vi "Filter And List Splitters.vi"(8 "Error In":errorcluster, 10 "Splitter Refs":refnum<vi>[](array[refnum]), 11 "Control Reference Lists In":T1) -> (0 "Error Out":errorcluster, 3 "Control Reference Lists Out":T1)   [LabVIEW 2021, in "Appearance Actor.lvlib" / "Appearance Actor.lvclass"]
uses:
  Appearance Actor.lvclass
  Typedefs/Control Reference Lists--cluster.ctl
  Typedefs/Control Reference Lists-TitleBar--cluster.ctl
  Typedefs/Control Reference Lists-SideMenu--cluster.ctl
  Typedefs/Control Reference Lists-BodyPane--cluster.ctl
  Typedefs/Control Reference Lists-StatusBar--cluster.ctl
  <vilib>/regexp/Match Regular Expression.xnode
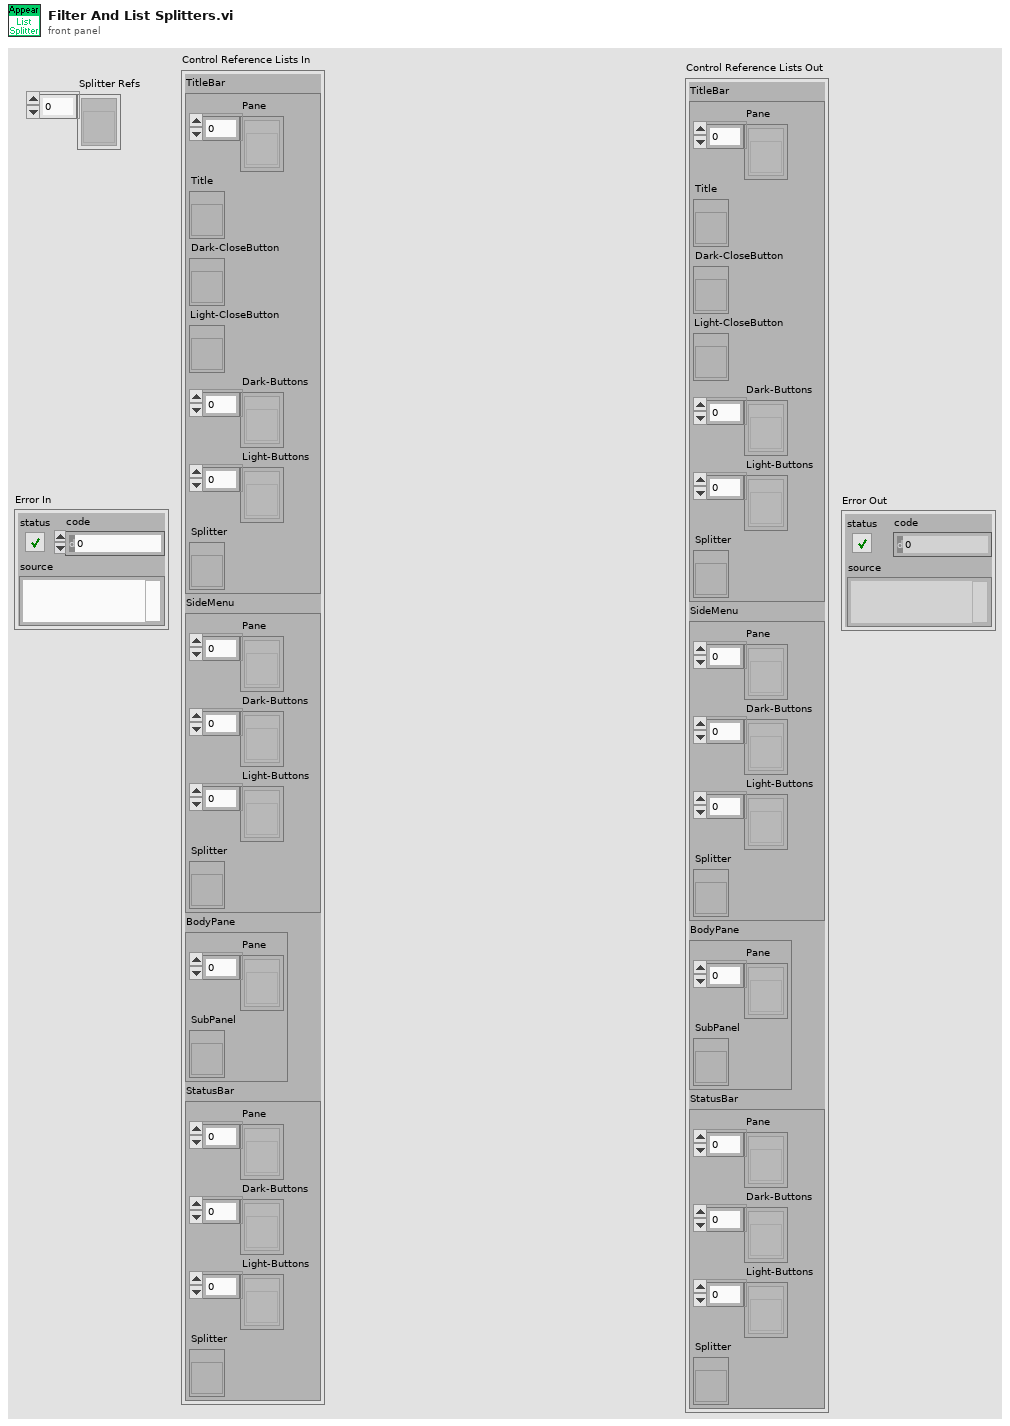
[diagram p1: front panel]
types:
  T1 = typedef "Control Reference Lists--cluster.ctl" = cluster{"TitleBar":T2, "SideMenu":T3, "BodyPane":T4, "StatusBar":T5}
  T2 = typedef "Control Reference Lists-TitleBar--cluster.ctl" = cluster{"Pane":refnum<vi>[], "Title":refnum<vi>, "Dark-CloseButton":refnum<vi>, "Light-CloseButton":refnum<vi>, "Dark-Buttons":refnum<vi>[], "Light-Buttons":refnum<vi>[], "Splitter":refnum<vi>}
  T3 = typedef "Control Reference Lists-SideMenu--cluster.ctl" = cluster{"Pane":refnum<vi>[], "Dark-Buttons":refnum<vi>[], "Light-Buttons":refnum<vi>[], "Splitter":refnum<vi>}
  T4 = typedef "Control Reference Lists-BodyPane--cluster.ctl" = cluster{"Pane":refnum<vi>[], "SubPanel":refnum<vi>}
  T5 = typedef "Control Reference Lists-StatusBar--cluster.ctl" = cluster{"Pane":refnum<vi>[], "Dark-Buttons":refnum<vi>[], "Light-Buttons":refnum<vi>[], "Splitter":refnum<vi>}
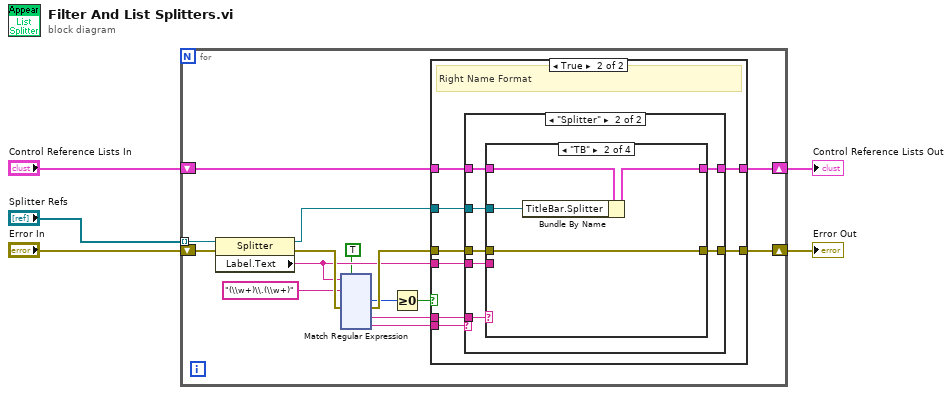
[diagram p0: block diagram]
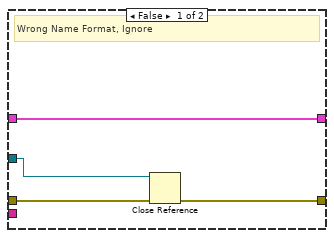
[diagram p2: hidden frame]
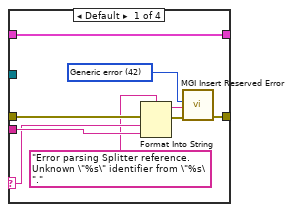
[diagram p4: hidden frame]
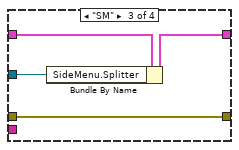
[diagram p5: hidden frame]
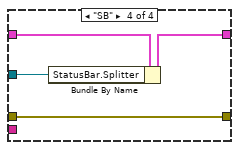
[diagram p6: hidden frame]
diagram:
  n1 = for {
    tunnel: "Splitter Refs" -> [w20] mode=indexing
    shift-right: [w12] -> w1
    shift-left: "Error In" -> [w19]
    shift-right: [w15] -> w2
    shift-left: "Control Reference Lists In" -> [w17]
    n2 = property class="Splitter"(reference=w20, error in=w19) -> (reference out=w14:refnum<vi>, error out=w18:errorcluster, "Label.Text"=w10:string)
    n3 = xnode "Match Regular Expression"("input string"=w10, "regular expression"="(\\w+)\\.(\\w+)", "error in"=w18, "ignore case? (F)"=TRUE) -> ("offset past match"=w7:i32, "error out"=w13:errorcluster, "submatch 1"=w16:string, "submatch 2"=w8:string)  [unwired: 2 in, 3 out]
    n4 = Greater Or Equal To 0?(x=w7) -> (x >= 0?=w6:bool)
    n5 = case shown="True" w6 {
      tunnel: w17 -> [w24 w32]
      tunnel: w16 -> [_ w31]
      tunnel: [w24 w30] -> w15
      tunnel: w14 -> [w21 w29]
      tunnel: w13 -> [w23 w28]
      tunnel: [w22 w27] -> w12
      tunnel: w10 -> [_ w26]
      tunnel: w8 -> [_ w25]
      frame False {
        # "Wrong Name Format, Ignore"
        n6 = Close Reference(reference=w21, error in (no error)=w23) -> (error out=w22:errorcluster)
      }
      frame True {
        # "Right Name Format"
        n7 = case shown="\"Splitter\"" w25 {
          tunnel: w32 -> [w33 w41]
          tunnel: w31 -> [_ w40]
          tunnel: [w33 w39] -> w30
          tunnel: w29 -> [_ w38]
          tunnel: w28 -> [w34 w37]
          tunnel: [w34 w36] -> w27
          tunnel: w26 -> [_ w35]
          frame Default {
            # "Can be subsplitter, allow"
            # "SubSplitter or other"
          }
          frame "Splitter" {
            # "Splitter"
            n8 = case shown="\"TB\"" w40 {
              selector: w40 -> [w43 _ _ _]
              tunnel: w41 -> [w50 w54 w58 w62]
              tunnel: [w50 w53 w57 w61] -> w39
              tunnel: w38 -> [_ w52 w56 w60]
              tunnel: w37 -> [w46 w51 w55 w59]
              tunnel: [w45 w51 w55 w59] -> w36
              tunnel: w35 -> [w44 _ _ _]
              frame Default {
                w47 = 42 items=["No error", "Argument error", "Memory is full", "Out of zone", "End of file", "File already open", "Generic file I/O error", "File not found", "File permission error", "Disk is full", "Duplicate path", "Too many files open", "System feature not enabled", "Resource file not found", "Cannot add resource", "Resource not found", "Image not found", "Image memory error", "Pen does not exist", "Config type invalid", "Config token not found", "Config parse error", "Config memory error", "Bad external code format", "Bad external code offset", "External code not present", "Null window", "Destroy window error", "Null menu", "Print aborted", "Bad print record", "Print driver error", "Windows error during printing", "Memory error during printing", "Print dialog error", "Generic print error", "Invalid device refnum", "Device not found", "Device parameter error", "Device unit error", "Cannot open device", "Device call aborted", "Generic error", "Cancelled by user", "Object ID too low", "Object ID too high", "Object not in heap", "Unknown heap", "Unknown object (invalid DefProc)", "Unknown object (DefProc not in table)", "Message out of range", "Invalid (null) method", "Unknown message", "Manager call not supported", "Bad address", "Network operation in progress", "Network operation timed out", "Connection is busy", "Network attribute not supported", "Network error", "Address in use", "System out of memory", "Connection aborted", "Connection refused", "Not connected", "Already connected", "Connection closed", "Initialization error (interapplication manager)", "Bad occurrence", "Wait on unbound occurrence handler", "Occurrence queue overflow", "Datalog type conflict", "Unused", "Unrecognized type (interapplication manager)", "Memory corrupt", "Failed to make temporary DLL", "Old CIN version", "Drag socket not found", "Failed to load drop-object", "Failed to register OLE object", "Failed to release OLE object", "Format specifier type mismatch", "Unknown format specifier", "Too few format specifiers", "Too many format specifiers", "Scan failed", "Newer CIN version", "OLE Convert", "Runtime menu error", "Password tampered", "Unknown error code"] ("Reserved Error Code (Generic error)")
                n9 = Format Into String(format string="Error parsing Splitter reference. Unknown \"%s\" identifier from \"%s\".", error in=w46, w43, w44) -> (resulting string=w49:string, error out=w48:errorcluster)  [unwired: 1 in]
                n10 = call <userlib>:"MGI Insert Reserved Error.vi"("Error In"=w48, "Error Description"=w49, "Reserved Error Code (Generic error)"=w47) -> ("Error Out"=w45:errorcluster)  [unwired: 8 in]
              }
              frame "TB" {
                n11 = Bundle By Name(cluster=w54, "TitleBar.Splitter"=w52) -> (w53:T1)
              }
              frame "SM" {
                n12 = Bundle By Name(cluster=w58, "SideMenu.Splitter"=w56) -> (w57:T1)
              }
              frame "SB" {
                n13 = Bundle By Name(cluster=w62, "StatusBar.Splitter"=w60) -> (w61:T1)
              }
            }
          }
        }
      }
    }
  }
  "Error Out" <- w1
  "Control Reference Lists Out" <- w2
